vi "Start_Client.vi"   [LabVIEW 2020]
uses:
  Database/Global1.vi
types:
  T1 = cluster{"设备名称":string, "操作人员":string, "设备状态":enum16{"设备离线", "设备正常", "设备缺料", "设备故障", "质量报警"}, "附加信息":string}
  T2 = enum32{"Invalid", "Standard", "Closed", "Hidden", "Minimized", "Maximized"}
  T3 = cluster{"用户编号":string, "用户名":string, "用户密码(密文)":string, "用户权限":string}
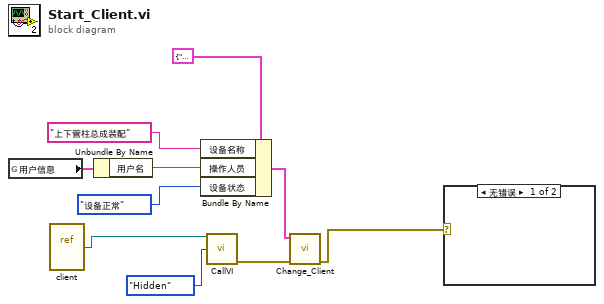
[diagram p0: block diagram]
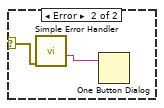
[diagram p2: hidden frame]
diagram:
  n1 = global read "Global1.vi" "用户信息"() -> (w3:T3)
  n2 = vi-ref "client.vi"() -> (w1:refnum<vi>)
  n3 = Unbundle By Name(w3) -> ("用户名"=w5:string)
  n4 = Bundle By Name(cluster=T1 {"设备名称"="", "操作人员"="", "设备状态"=enum."设备离线", "附加信息"=""} ("设备信息"), "设备名称"="上下管柱总成装配", "操作人员"=w5, "设备状态"=enum16{"设备离线", "设备正常", "设备缺料", "设备故障", "质量报警"}."设备正常") -> (w4:T1)
  n5 = call "CallVI.vi"("VI引用"=w1, "状态"=T2."Hidden") -> ("错误输出"=w9:errorcluster)  [unwired: 11 in, 2 out]
  n6 = call "Change_Client.vi"("错误输入（无错误）"=w9, "设备信息"=w4) -> ("错误输出"=w2:errorcluster)  [unwired: 9 in]
  n7 = case shown="无错误" w2 {
    selector: w2 -> [_ w11]
    frame No Error {
    }
    frame Error {
      n8 = call <vilib>:"Simple Error Handler.vi"("error in (no error)"=w11) -> ("source out"=w12:string)  [unwired: 4 in, 4 out]
      n9 = One Button Dialog(message=w12) -> ()  [unwired: 1 in, 1 out]
    }
  }
